vi "Run.vi"(8 "error in (no error)":errorcluster caption="entrée d'erreur (pas d'erreur)", 9 "X":string[][](array[string]), 10 "Type X":T1(ring), 11 "scale.lvclass":refnum<class "scale.lvclass">) -> (0 "error out":errorcluster caption="sortie d'erreur", 2 "Data":T2, 3 "scale.lvclass":refnum<class "scale.lvclass">)   [LabVIEW 2020, in "scale.lvclass"]
uses:
  scale.lvclass
  scale.lvclass/scale.ctl
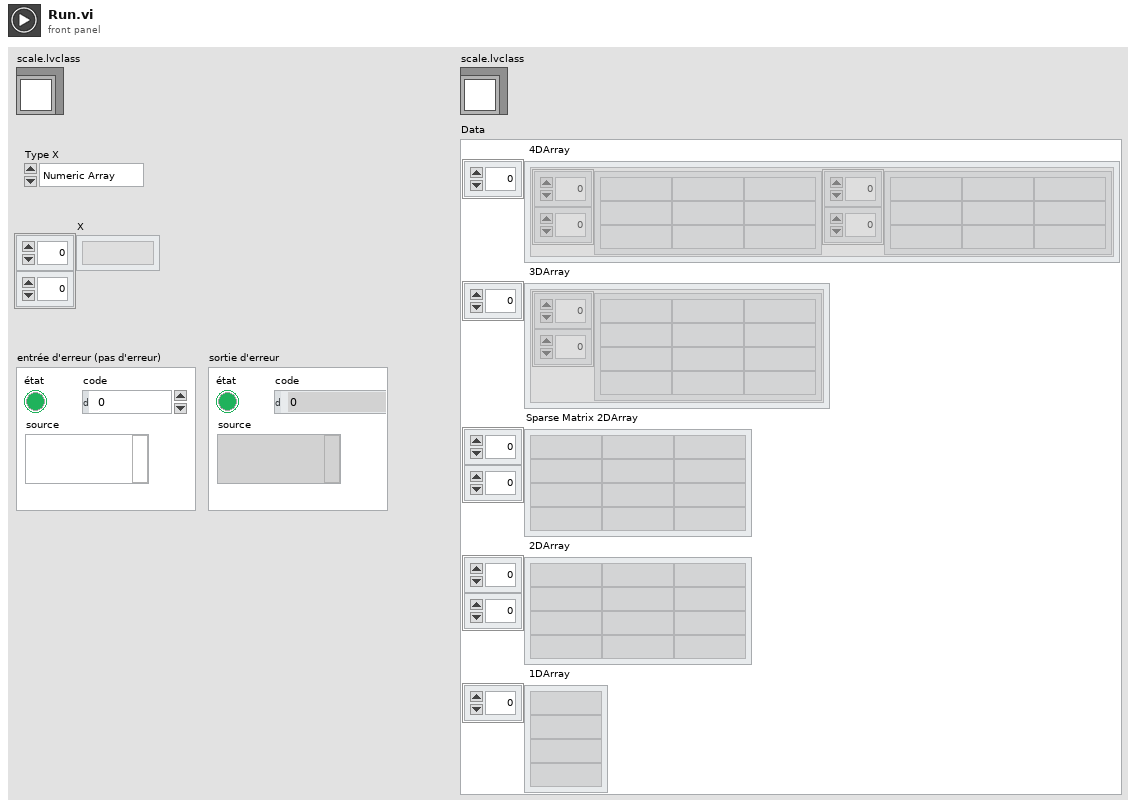
[diagram p1: front panel]
types:
  T1 = enum16{"Numeric Array", "String Array", "Sparse"}
  T2 = cluster{" 4DArray":cluster{"1":string[][], "2":string[][]}[], " 3DArray":cluster{"Tableau":string[][]}[], "Sparse Matrix 2DArray":string[][], " 2DArray":string[][], " 1DArray":string[]}
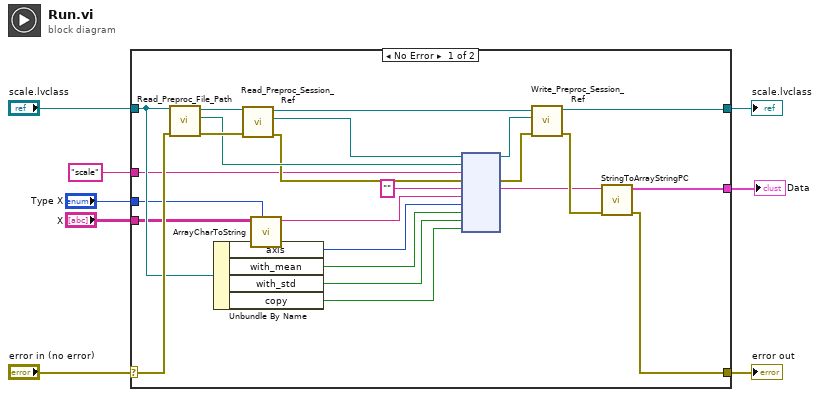
[diagram p0: block diagram]
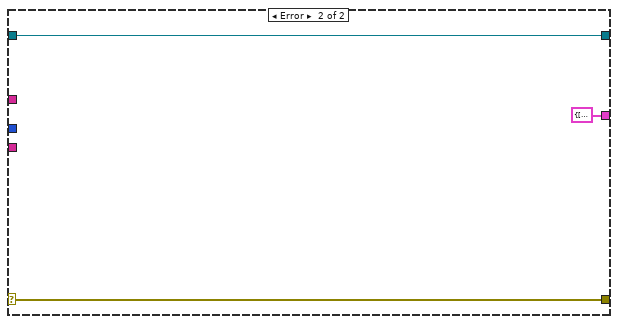
[diagram p2: hidden frame]
diagram:
  n1 = case shown="No Error" "error in (no error)" {
    selector: "error in (no error)" -> [w21 w35]
    tunnel: [w10 w35] -> w7
    tunnel: [w13 w34] -> w5
    tunnel: "scale.lvclass" -> [w20 w34]
    tunnel: "scale" ("Fonction") -> [w19 _]
    tunnel: [w9 T2 {" 4DArray"=[], " 3DArray"=[], "Sparse Matrix 2DArray"=[], " 2DArray"=[], " 1DArray"=[]} ("Data")] -> w1
    tunnel: "X" -> [w15 _]
    tunnel: "Type X" -> [w16 _]
    frame No Error {
      n2 = call-dynamic "Read_Preproc_File_Path.vi"("error in (no error)"=w21, "Python in"=w20) -> ("error out"=w31:errorcluster, "File_Path"=w28:path, "Python out"=w32:refnum<class "scale.lvclass">)  [unwired: 7 in]
      n3 = Unbundle By Name(w20) -> ("axis"=w23:i32, "with_mean"=w22:bool, "with_std"=w18:bool, "copy"=w17:bool)
      n4 = call-dynamic "Read_Preproc_Session_Ref.vi"("error in (no error)"=w31, "Python in"=w32) -> ("error out"=w27:errorcluster, "Session_ref"=w29:refnum<k35>, "Python out"=w30:refnum<class "scale.lvclass">)  [unwired: 7 in]
      n5 = call "ArrayCharToString.vi"("Type"=w16, "TAB"=w15) -> ("Instruction"=w14:string)  [unwired: 9 in]
      n6 = node(w29, w28, w19, w27, "", w14, w23, w22, w18, w17) -> (w25:refnum<k35>, w26:errorcluster, w11:string)  [unwired: 5 in, 2 out]
      n7 = call-dynamic "Write_Preproc_Session_Ref.vi"("error in (no error)"=w26, "Session_ref"=w25, "Python in"=w30) -> ("error out"=w12:errorcluster, "Python out"=w13:refnum<class "scale.lvclass">)  [unwired: 7 in]
      n8 = call "StringToArrayStringPC.vi"("sortie d'erreur"=w12, "Return value"=w11) -> ("sortie d'erreur"=w10:errorcluster, "Data"=w9:T2)  [unwired: 8 in]
    }
    frame Error {
    }
  }
  "error out" <- w7
  "scale.lvclass" <- w5
  "Data" <- w1
